vi "Advance past colon.vi"(7 "JSON":string, 9 "Offset":i32, 11 "State":T1=enum."Leading Whitespace") -> (1 "index":i32, 3 "State":T1=enum."Value end")   [LabVIEW 2015, in "JSONtext.lvlib"]
uses:
  JSONtext.lvlib
  Parsing State.ctl
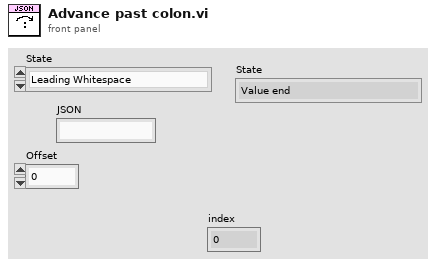
[diagram p1: front panel]
types:
  T1 = typedef "JSONtext.lvlib/Parsing State.ctl" = enum16{"Parser Error", "Object", "Array", "String", "Number/Other", "Leading Whitespace", "Object end", "Array end", "Value end"}
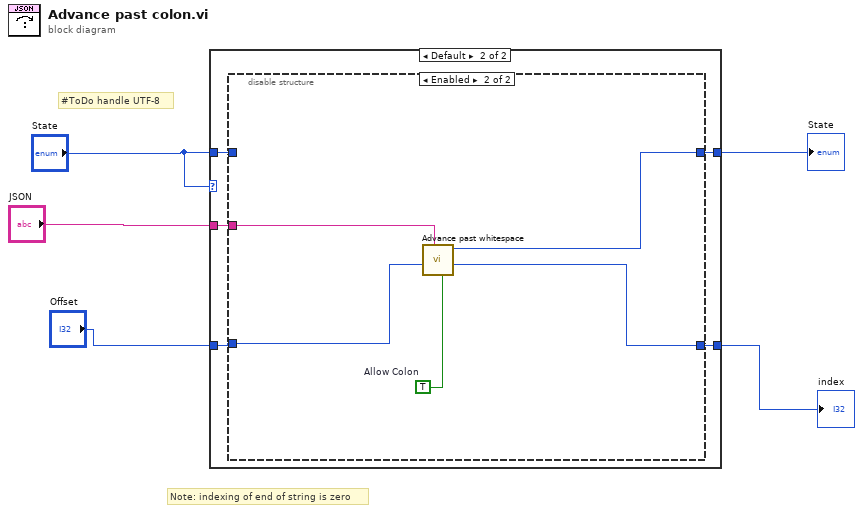
[diagram p0: block diagram]
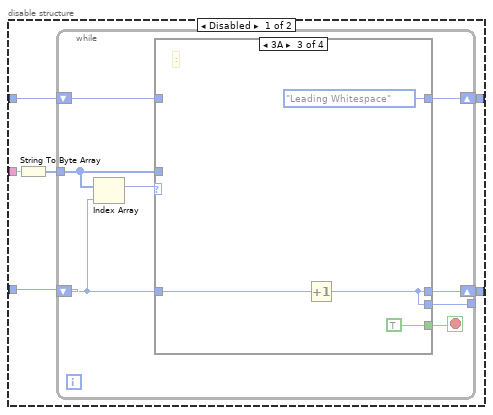
[diagram p3: hidden frame]
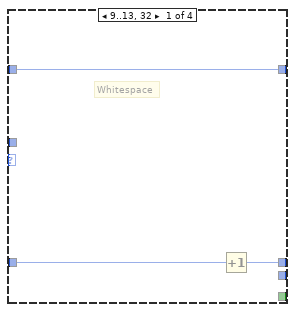
[diagram p4: hidden frame]
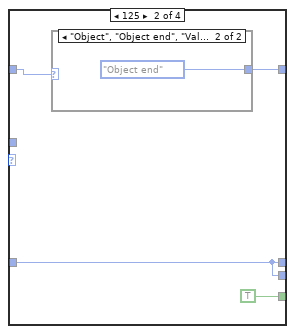
[diagram p5: hidden frame]
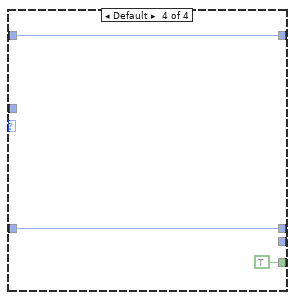
[diagram p7: hidden frame]
diagram:
  # "Note: indexing of end of string is zero"
  # "#ToDo handle UTF-8"
  n1 = case shown="Default" "State" {
    tunnel: [w7 w12] -> w5
    tunnel: [w6 w11] -> w4
    tunnel: "State" -> [w7 w10]
    tunnel: "Offset" -> [w6 w9]
    tunnel: "JSON" -> [_ w8]
    frame "Parser Error" {
    }
    frame Default {
      n2 = disable-structure shown="Enabled" {
        disable-tunnel: [w18 w42] -> w12
        disable-tunnel: [w17 w43] -> w11
        disable-tunnel: w10 -> [w16 _]
        disable-tunnel: w9 -> [w15 w44]
        disable-tunnel: w8 -> [w14 w46]
        frame Disabled {
          n3 = String To Byte Array(string=w14) -> (unsigned byte array=w13:u8[])
          n4 = while {
            tunnel: w13 -> [w25]
            shift-right: [w20] -> w17
            shift-left: w15 -> [w21]
            shift-right: [w23] -> w18
            shift-left: w16 -> [w24]
            tunnel: [w19] -> _
            stop <- w22 stop-if-true
            n5 = Index Array(array=w25, index=w21) -> (element=w26:u8)
            n6 = case shown="3A" w26 {
              tunnel: w25 -> [_ _ _ _]
              tunnel: w24 -> [w29 w30 _ w39]
              tunnel: [w29 w33 Parsing_State."Leading Whitespace" w39] -> w23
              tunnel: [_ TRUE TRUE TRUE] -> w22
              tunnel: w21 -> [w28 w31 w37 w41]
              tunnel: [w27 w31 w35 w41] -> w20
              tunnel: [_ w31 w35 _] -> w19
              frame 9..13, 32 {
                # "Whitespace"
                n7 = Increment(x=w28) -> (x+1=w27:i32)
              }
              frame 125 {
                n8 = case shown="\"Object\", \"Object end\", \"Value end\"" w30 {
                  tunnel: [_ Parsing_State."Object end"] -> w33
                  frame Default {
                  }
                  frame "Object", "Object end", "Value end" {
                  }
                }
              }
              frame 58 {
                # ":"
                n9 = Increment(x=w37) -> (x+1=w35:i32)
              }
              frame Default {
              }
            }
          }
        }
        frame Enabled {
          w45 = TRUE  # Allow Colon
          n10 = call "Advance past whitespace.vi"("Past Colon"=w45, "JSON"=w46, "Offset"=w44) -> ("Offset of first non-whitespace"=w43:i32, "Parser State"=w42:T1)  [unwired: 7 in]
        }
      }
    }
  }
  "State" <- w5
  "index" <- w4
